vi "Check Local Msg Set.vi"(10 "Msg":refnum<class "Msg.lvclass">, 11 "TEMPLATE Actor in":refnum<class "TEMPLATE Actor.lvclass">) -> (0 "Error out":errorcluster, 3 "TEMPLATE Actor out":refnum<class "TEMPLATE Actor.lvclass">)   [LabVIEW 2020, in "_Template.lvlib" / "Templates.lvlib" / "TEMPLATE Actor.lvlib" / "TEMPLATE Actor.lvclass"]
uses:
  TEMPLATE Actor.lvclass
  C:/git/jettl/src/jettl/jettl/Actor/Actor/Actor.lvclass
  jettl/jettl/Msg/Msg.lvclass
  TEMPLATE Actor.lvclass/TEMPLATE Actor.ctl
  jettl/jettl/Actor/Actor/Actor.lvclass
  jettl/jettl/Actor/Actor.lvlib
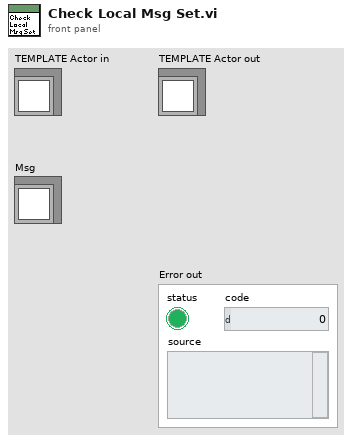
[diagram p1: front panel]
types:
  T1 = typedef "jettl.lvlib/Actor.lvlib/Msg Set.ctl" = set{refnum<class "Msg.lvclass">}
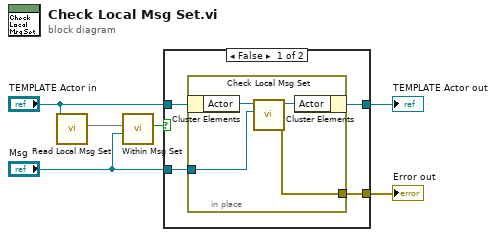
[diagram p0: block diagram]
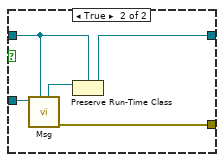
[diagram p2: hidden frame]
diagram:
  n1 = call-dynamic "Read Local Msg Set.vi"("TEMPLATE Actor in"="TEMPLATE Actor in") -> ("Local Msg Set"=w1:T1)  [unwired: 10 in]
  n2 = call "Within Msg Set.vi"("Msg"="Msg", "Msg Set"=w1) -> ("Within Msg Set"=w6:bool)  [unwired: 9 in]
  n3 = case shown="False" w6 {
    tunnel: "TEMPLATE Actor in" -> [w10 w17]
    tunnel: [w9 w16] -> w5
    tunnel: "Msg" -> [w8 w19]
    tunnel: [w7 w15] -> w3
    frame False {
      n4 = in-place {
        in-place-border: w8 -> [w12]
        in-place-border: [w11] -> w7
        n5 = in-place-cluster #1(w10) -> ("Actor"=w14:refnum<class "Actor.lvclass">)
        n6 = call-dynamic "Check Local Msg Set.vi"("Msg"=w12, "Actor in"=w14) -> ("Error out"=w11:errorcluster, "Actor out"=w13:refnum<class "Actor.lvclass">)  [unwired: 8 in]
        n7 = in-place-cluster #1("Actor"=w13) -> (w9:refnum<class "TEMPLATE Actor.lvclass">)
      }
    }
    frame True {
      n8 = call-dynamic "Msg.vi"("Actor in"=w17, "Msg in"=w19) -> ("Error out"=w15:errorcluster, "Actor out"=w18:refnum<class "Actor.lvclass">)  [unwired: 8 in]
      n9 = Preserve Run-Time Class(object in=w18, 2:w17) -> (object out=w16:refnum<class "TEMPLATE Actor.lvclass">)  [unwired: 1 in, 1 out]
    }
  }
  "TEMPLATE Actor out" <- w5
  "Error out" <- w3
